vi "remote.Write client handle.vi"(8 "error in (no error)":errorcluster, 10 "Client Handle":T1, 11 "SLSC Remote in":refnum<class "SLSC Remote.lvclass">) -> (0 "error out":errorcluster, 3 "SLSC Remote out":refnum<class "SLSC Remote.lvclass">)   [LabVIEW 2016, in "SLSC Remote.lvclass"]
uses:
  SLSC Remote.lvclass
  <vilib>/httpClient/ClientHandle.ctl
  <vilib>/httpClient/LabVIEWHTTPClient.lvlib
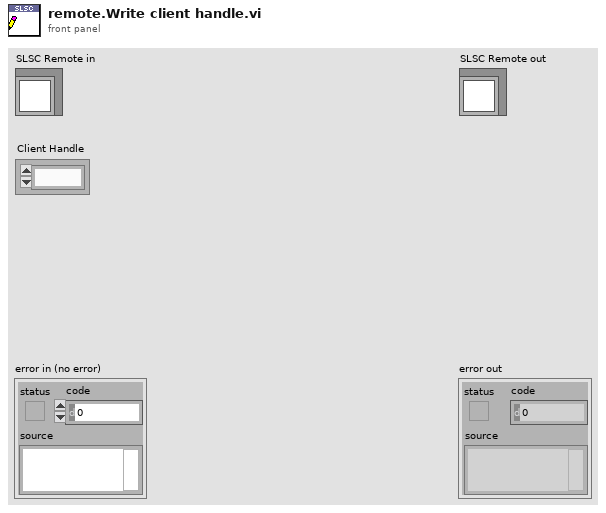
[diagram p1: front panel]
types:
  T1 = typedef "LabVIEWHTTPClient.lvlib/ClientHandle.ctl" = refnum<k1>
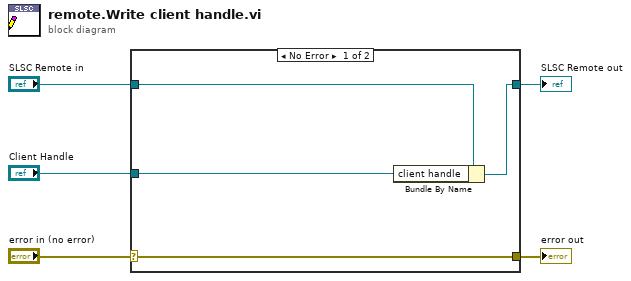
[diagram p0: block diagram]
diagram:
  n1 = case shown="No Error" "error in (no error)" {
    selector: "error in (no error)" -> [w9 w10]
    tunnel: [w9 w10] -> w4
    tunnel: [w7 w11] -> w2
    tunnel: "SLSC Remote in" -> [w8 w11]
    tunnel: "Client Handle" -> [w6 _]
    frame No Error {
      n2 = Bundle By Name(cluster=w8, "client handle"=w6) -> (w7:refnum<class "SLSC Remote.lvclass">)
    }
    frame Error {
    }
  }
  "error out" <- w4
  "SLSC Remote out" <- w2
